vi "SendQuery.vi"(8 "error in (no error)":errorcluster, 11 "TCPComm in":refnum<class "TCPCommClass.lvclass">) -> (0 "error out":errorcluster, 3 "TCPComm out":refnum<class "TCPCommClass.lvclass">)   [LabVIEW 2013, in "TCPCommClass.lvclass"]
uses:
  TCPCommClass.lvclass
  TCPCommClass.lvclass/TCPCommClass.ctl
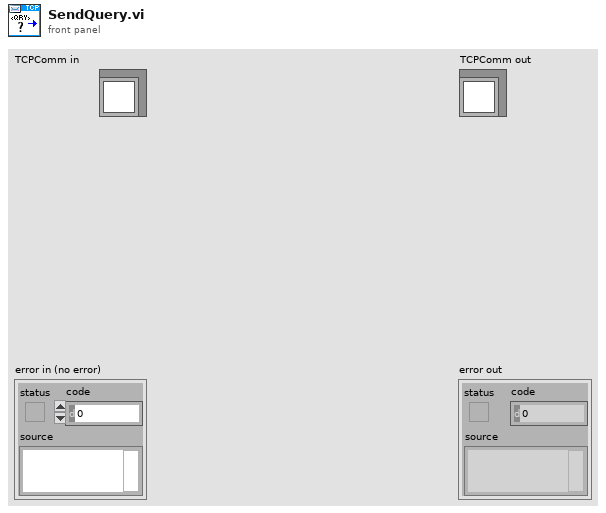
[diagram p1: front panel]
types:
  T1 = enum16{"Standard", "Buffered", "CRLF", "Immediate"}
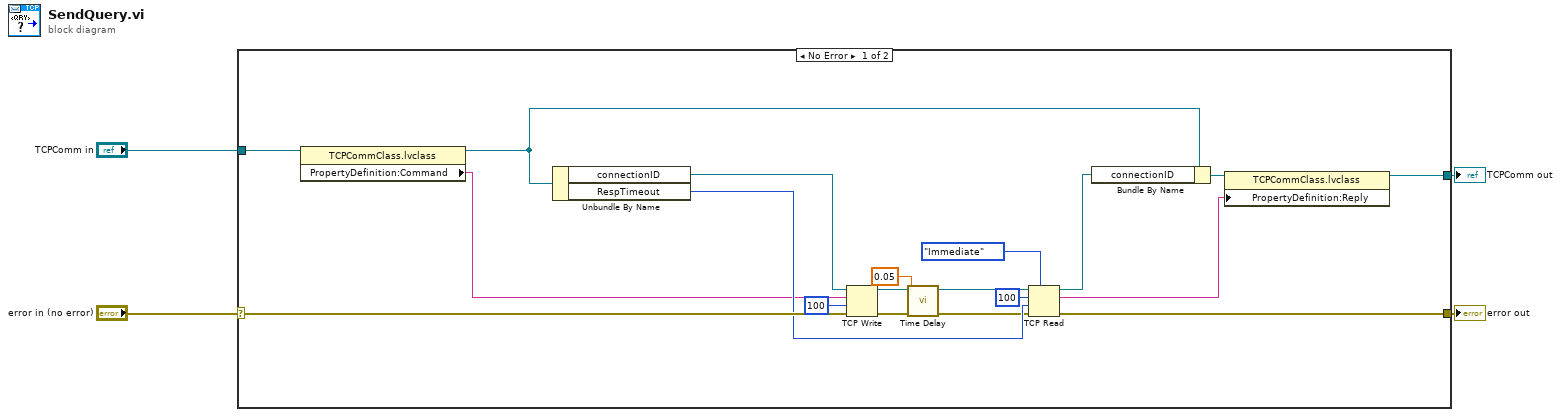
[diagram p0: block diagram]
diagram:
  n1 = case shown="No Error" "error in (no error)" {
    selector: "error in (no error)" -> [w18 w24]
    tunnel: [w17 w24] -> w3
    tunnel: [w10 w23] -> w1
    tunnel: "TCPComm in" -> [w13 w23]
    frame No Error {
      n2 = property class="TCPCommClass.lvclass"(reference=w13) -> (reference out=w12:refnum<class "TCPCommClass.lvclass">, "PropertyDefinition:Command"=w8:string)  [unwired: 1 in, 1 out]
      n3 = Unbundle By Name(w12) -> ("connectionID"=w15:refnum<k5>, "RespTimeout"=w14:i32)
      n4 = TCP Write(connection ID=w15, data in=w8, error in (no error)=w18, 9:100 ("bytes to read")) -> (connection ID out=w21:refnum<k5>, error out=w22:errorcluster)  [unwired: 1 out]
      n5 = call "Time Delay"("error in (no error)"=w22, "Delay Time (s)"=0.05) -> ("error out"=w6:errorcluster)  [unwired: 9 in]
      n6 = TCP Read(connection ID=w21, bytes to read=100, error in (no error)=w6, 7:T1."Immediate" ("mode (standard)"), 9:w14) -> (connection ID out=w16:refnum<k5>, data out=w9:string, error out=w17:errorcluster)
      n7 = Bundle By Name(cluster=w12, "connectionID"=w16) -> (w11:refnum<class "TCPCommClass.lvclass">)
      n8 = property class="TCPCommClass.lvclass"(reference=w11, "PropertyDefinition:Reply"=w9) -> (reference out=w10:refnum<class "TCPCommClass.lvclass">)  [unwired: 1 in, 1 out]
    }
    frame Error {
    }
  }
  "error out" <- w3
  "TCPComm out" <- w1
